vi "AlliGator Add Average Lifetime to Plot.vi"(5 "New Plot Name":string, 7 "Plot ID (-1)":i32=-1, 8 "error in (no error)":errorcluster, 9 "Average Lifetime":dbl, 10 "Abscissa":dbl, 11 "Lifetime Graph refnum":refnum<vi>) -> (0 "error out":errorcluster, 1 "# Plots":i32, 2 "Actual Plot ID":i32, 3 "Average Lifetime (dup)":dbl)   [LabVIEW 2021, in "AlliGator Lifetime.lvlib"]
doc: "Adds a single lifetime data point to a plot."
uses:
  AlliGator Lifetime.lvlib
  Graphs/XY Graph/XY Graph Add-Ons.lvlib
panel:
  # "see the AlliGator License on the block diagram (Ctrl+E or Window:Show Block Diagram)"
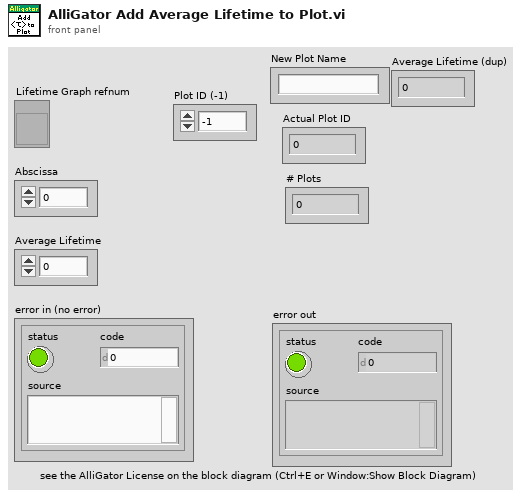
[diagram p1: front panel]
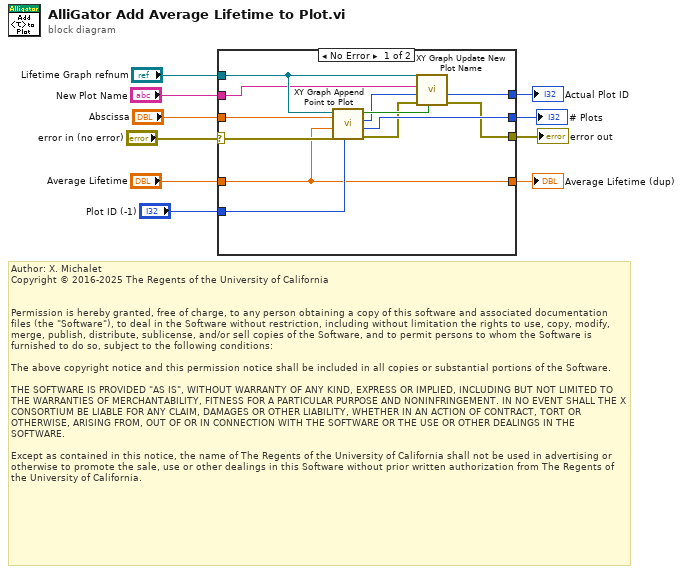
[diagram p0: block diagram]
diagram:
  # "Author: X. Michalet\nCopyright © 2016-2025 The Regents of the University of California\n \n\nPermission is hereby granted, free of charge, to any person obtaining a copy of this software and associated documentation files (the \"Software\"), to deal in the Software without restriction, including without limitation the rights to use, copy, modify, merge, publish, distribute, sublicense, and/or sell copies of the Software, and to permit persons to whom the Software is furnished to do so, subject to the following conditions:\n\nThe above copyright notice and this permission notice shall be included in all copies or substantial portions of the Software.\n\nTHE SOFTWARE IS PROVIDED \"AS IS\", WITHOUT WARRANTY OF ANY KIND, EXPRESS OR IMPLIED, INCLUDING BUT NOT LIMITED TO THE WARRANTIES OF MERCHANTABILITY, FITNESS FOR A PARTICULAR PURPOSE AND NONINFRINGEMENT. IN NO EVENT SHALL THE X CONSORTIUM BE LIABLE FOR ANY CLAIM, DAMAGES OR OTHER LIABILITY, WHETHER IN AN ACTION OF CONTRACT, TORT OR OTHERWISE, ARISING FROM, OUT OF OR IN CONNECTION WITH THE SOFTWARE OR THE USE OR OTHER DEALINGS IN THE SOFTWARE.\n\nExcept as contained in this notice, the name of The Regents of the University of California shall not be used in advertising or otherwise to promote the sale, use or other dealings in this Software without prior written authorization from The Regents of the University of California."
  n1 = case shown="No Error" "error in (no error)" {
    selector: "error in (no error)" -> [w21 w23]
    tunnel: "Average Lifetime" -> [w11 w22]
    tunnel: [w13 w23] -> w8
    tunnel: "Plot ID (-1)" -> [w20 _]
    tunnel: [w19 _] -> w6
    tunnel: [w15 _] -> w5
    tunnel: "Lifetime Graph refnum" -> [w17 _]
    tunnel: "New Plot Name" -> [w16 _]
    tunnel: [w11 w22] -> w2
    tunnel: "Abscissa" -> [w12 _]
    frame No Error {
      n2 = call "XY Graph Append Point to Plot.vi"("Plot ID (-1: last)"=w20, "error in (no error)"=w21, "y"=w11, "x"=w12, "XYGraph in"=w17) -> ("error out"=w14:errorcluster, "# Plots"=w19:i32, "Actual Plot ID"=w15:i32, "Plot Created?"=w18:bool)  [unwired: 3 in]
      n3 = call "XY Graph Update New Plot Name.vi"("Plot Created?"=w18, "error in (no error)"=w14, "Actual Plot ID"=w15, "New Plot Name"=w16, "XYGraph in"=w17) -> ("error out"=w13:errorcluster)  [unwired: 6 in]
    }
    frame Error {
    }
  }
  "error out" <- w8
  "# Plots" <- w6
  "Actual Plot ID" <- w5
  "Average Lifetime (dup)" <- w2
